vi "Sub UI Plot Frame.vi"(8 "error in (no error)":errorcluster, 9 "frames":T2, 10 "Img Data indexed":cluster{"image data":T1, "bitmap":u32[][]}, 11 "LF2R IDE in":refnum<class "LF2R IDE.lvclass">) -> (0 "error out":errorcluster, 3 "LF2R IDE out":refnum<class "LF2R IDE.lvclass">)   [LabVIEW 2018, in "LF2R IDE.lvlib" / "LF2R IDE.lvclass"]
uses:
  LF2R IDE.lvclass
  Image Json Parser/Img Json Frames.ctl
  <vilib>/picture/picture.llb/imagedata.ctl
  LF2R IDE.lvclass/LF2R IDE.ctl
  Image/Image Process.lvclass
  Image Json Parser/Image Json Parser.lvclass
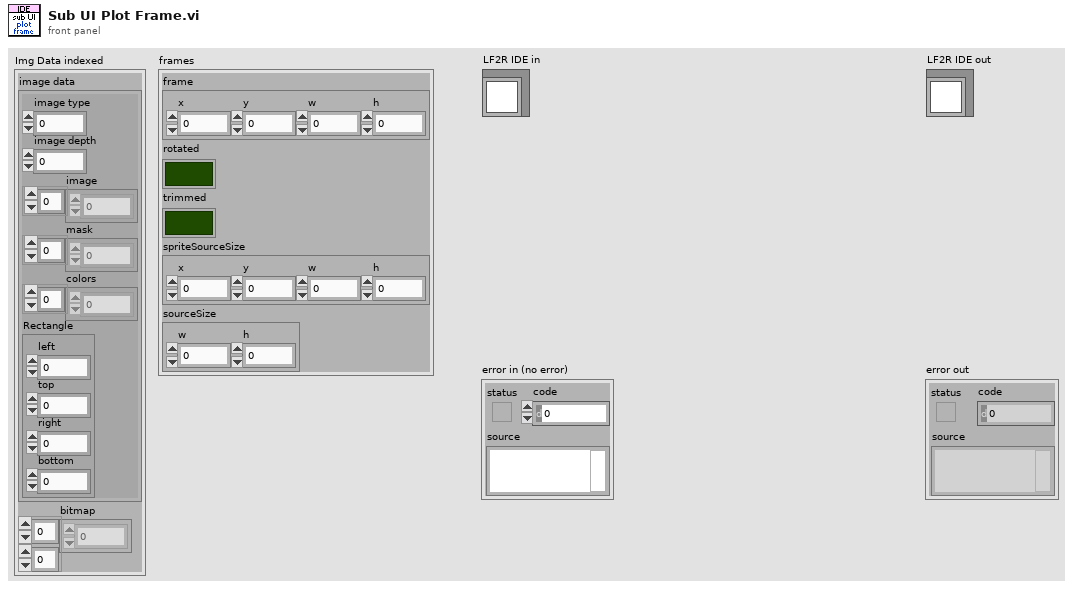
[diagram p1: front panel]
types:
  T1 = typedef "imagedata.ctl" = cluster{"image type":i32, "image depth":i32, "image":u8[], "mask":u8[], "colors":u32[], "Rectangle":cluster{"left":i16, "top":i16, "right":i16, "bottom":i16}}
  T2 = typedef "Image Json Parser.lvclass/Img Json Frames.ctl" = cluster{"frame":cluster{"x":i32, "y":i32, "w":i32, "h":i32}, "rotated":bool, "trimmed":bool, "spriteSourceSize":cluster{"x":i32, "y":i32, "w":i32, "h":i32}, "sourceSize":cluster{"w":i32, "h":i32}}
  T3 = cluster{"left":i16, "top":i16, "right":i16, "bottom":i16}
  T4 = typedef "IMAQ Image.ctl" = refnum<image>
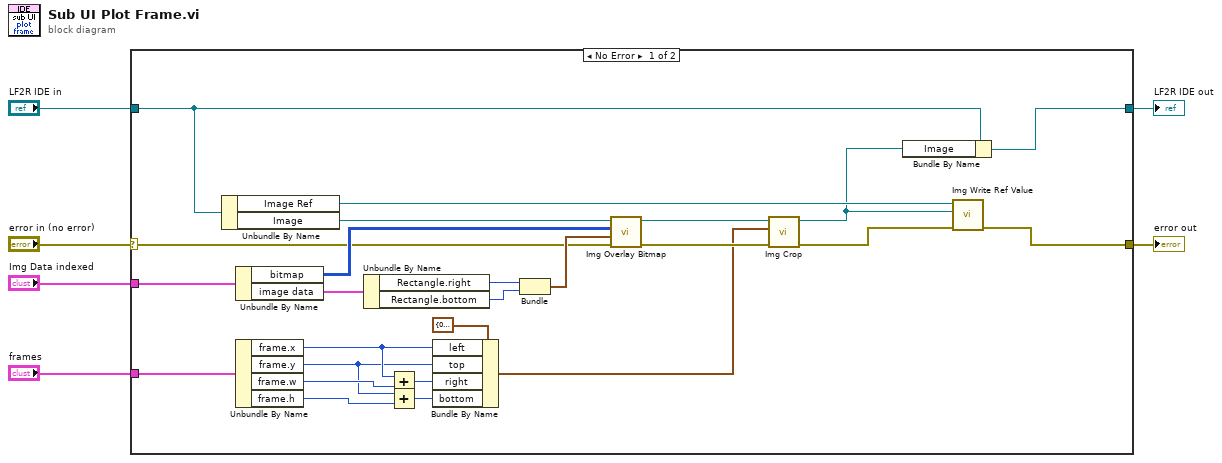
[diagram p0: block diagram]
diagram:
  n1 = case shown="No Error" "error in (no error)" {
    selector: "error in (no error)" -> [w13 w33]
    tunnel: [w10 w33] -> w5
    tunnel: [w8 w32] -> w3
    tunnel: "LF2R IDE in" -> [w12 w32]
    tunnel: "Img Data indexed" -> [w15 _]
    tunnel: "frames" -> [w14 _]
    frame No Error {
      n2 = Unbundle By Name(w12) -> ("Image Ref"=w9:refnum<vi>, "Image"=w16:T4)
      n3 = Unbundle By Name(w15) -> ("bitmap"=w22:u32[][], "image data"=w19:T1)
      n4 = Unbundle By Name(w14) -> ("frame.x"=w30:i32, "frame.y"=w27:i32, "frame.w"=w29:i32, "frame.h"=w25:i32)
      n5 = Unbundle By Name(w19) -> ("Rectangle.right"=w21:i16, "Rectangle.bottom"=w20:i16)
      n6 = Add(x=w30, y=w29) -> (x+y=w28:i32)
      n7 = Add(x=w27, y=w25) -> (x+y=w26:i32)
      n8 = Bundle By Name(cluster=T3 {"left"=0, "top"=0, "right"=269, "bottom"=269} ("Rectangle"), "left"=w30, "top"=w27, "right"=w28, "bottom"=w26) -> (w17:T3)
      n9 = Bundle("right"=w21, "bottom"=w20) -> (w18:cluster{"right":i16, "bottom":i16})  [unwired: 1 in]
      n10 = call "Img Overlay Bitmap.vi"("error in (no error)"=w13, "Size"=w18, "Bitmap"=w22, "Image"=w16) -> ("error out"=w23:errorcluster, "Image Out"=w24:T4)  [unwired: 6 in]
      n11 = call "Img Crop.vi"("error in (no error)"=w23, "Rectangle"=w17, "Image Src"=w24) -> ("error out"=w11:errorcluster, "Image Out"=w7:T4)  [unwired: 7 in]
      n12 = Bundle By Name(cluster=w12, "Image"=w7) -> (w8:refnum<class "LF2R IDE.lvclass">)
      n13 = call "Img Write Ref Value.vi"("error in (no error)"=w11, "Image"=w7, "Image Ref"=w9) -> ("error out"=w10:errorcluster)  [unwired: 8 in]
    }
    frame Error {
    }
  }
  "error out" <- w5
  "LF2R IDE out" <- w3
